vi "Update Position.vi"(8 "error in (no error)":errorcluster, 10 "Diff":cluster{"x":i16, "y":i16}, 11 "Line Border in":refnum<class "Line Border.lvclass">) -> (0 "error out":errorcluster, 1 "EndPoint":cluster{"x":i16, "y":i16}, 2 "StartPoint":cluster{"x":i16, "y":i16}, 3 "Line Border out":refnum<class "Line Border.lvclass">)   [LabVIEW 2015, in "Line Border.lvclass"]
uses:
  Line Border.lvclass
  Scalable Border/Scalable Border.lvclass/Scalable Border.ctl
  Line Border.lvclass/Line Border.ctl
  Scalable Border/Scalable Border.lvclass
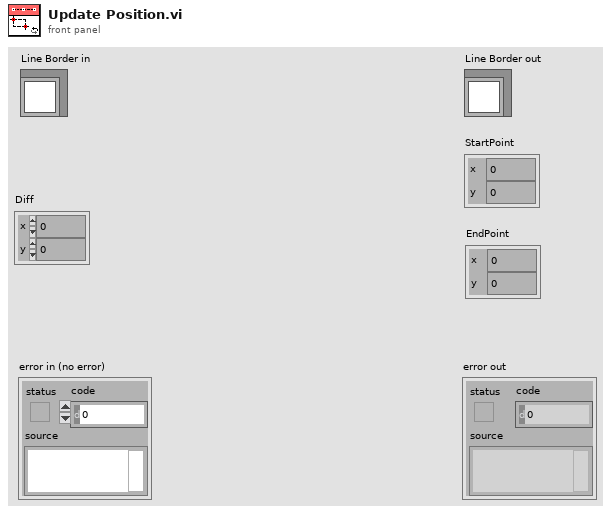
[diagram p1: front panel]
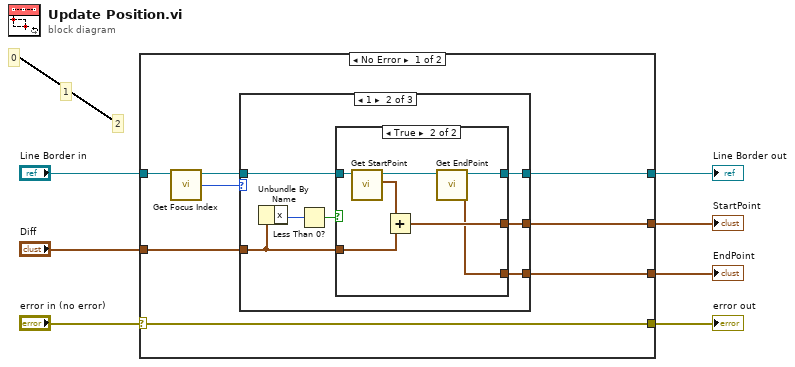
[diagram p0: block diagram]
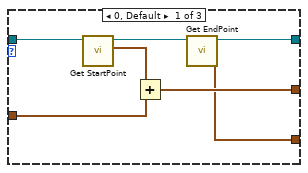
[diagram p2: hidden frame]
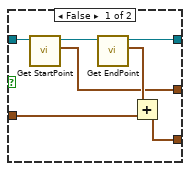
[diagram p3: hidden frame]
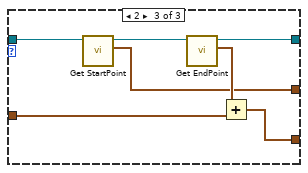
[diagram p4: hidden frame]
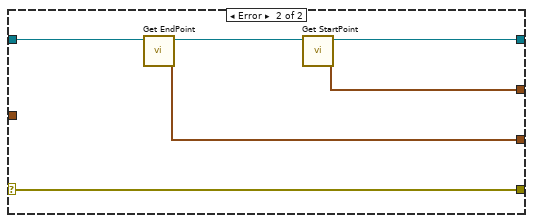
[diagram p5: hidden frame]
diagram:
  # "2"
  # "1"
  # "0"
  n1 = case shown="No Error" "error in (no error)" {
    selector: "error in (no error)" -> [w15 w56]
    tunnel: "Line Border in" -> [w14 w55]
    tunnel: [w11 w54] -> w5
    tunnel: "Diff" -> [w10 _]
    tunnel: [w9 w51] -> w3
    tunnel: [w8 w52] -> w2
    tunnel: [w15 w56] -> w1
    frame No Error {
      n2 = call "Get Focus Index.vi"("Scalable Border in"=w14) -> ("Focus Index"=w13:i8, "Scalable Border out"=w12:refnum<class "Line Border.lvclass">)  [unwired: 8 in, 1 out]
      n3 = case shown="1" w13 {
        tunnel: w12 -> [w22 w29 w50]
        tunnel: [w17 w27 w47] -> w11
        tunnel: w10 -> [w19 w25 w48]
        tunnel: [w18 w28 w44] -> w9
        tunnel: [w16 w26 w45] -> w8
        frame 0, Default {
          n4 = call "Get StartPoint.vi"("Line Border in"=w22) -> ("StartPoint"=w20:cluster{"x":i16, "y":i16}, "Line Border out"=w21:refnum<class "Line Border.lvclass">)  [unwired: 8 in, 1 out]
          n5 = Add(x=w20, y=w19) -> (x+y=w18:cluster{"x":i16, "y":i16})
          n6 = call "Get EndPoint.vi"("Line Border in"=w21) -> ("EndPoint"=w16:cluster{"x":i16, "y":i16}, "Line Border out"=w17:refnum<class "Line Border.lvclass">)  [unwired: 8 in, 1 out]
        }
        frame 1 {
          n7 = Unbundle By Name(w25) -> ("x"=w24:i16)
          n8 = Less Than 0?(x=w24) -> (x < 0?=w23:bool)
          n9 = case shown="True" w23 {
            tunnel: w29 -> [w34 w43]
            tunnel: [w32 w40] -> w28
            tunnel: [w33 w39] -> w27
            tunnel: [w30 w38] -> w26
            tunnel: w25 -> [w31 w37]
            frame False {
              n10 = call "Get StartPoint.vi"("Line Border in"=w34) -> ("StartPoint"=w32:cluster{"x":i16, "y":i16}, "Line Border out"=w36:refnum<class "Line Border.lvclass">)  [unwired: 8 in, 1 out]
              n11 = call "Get EndPoint.vi"("Line Border in"=w36) -> ("EndPoint"=w35:cluster{"x":i16, "y":i16}, "Line Border out"=w33:refnum<class "Line Border.lvclass">)  [unwired: 8 in, 1 out]
              n12 = Add(x=w35, y=w31) -> (x+y=w30:cluster{"x":i16, "y":i16})
            }
            frame True {
              n13 = call "Get StartPoint.vi"("Line Border in"=w43) -> ("StartPoint"=w41:cluster{"x":i16, "y":i16}, "Line Border out"=w42:refnum<class "Line Border.lvclass">)  [unwired: 8 in, 1 out]
              n14 = Add(x=w41, y=w37) -> (x+y=w40:cluster{"x":i16, "y":i16})
              n15 = call "Get EndPoint.vi"("Line Border in"=w42) -> ("EndPoint"=w38:cluster{"x":i16, "y":i16}, "Line Border out"=w39:refnum<class "Line Border.lvclass">)  [unwired: 8 in, 1 out]
            }
          }
        }
        frame 2 {
          n16 = call "Get StartPoint.vi"("Line Border in"=w50) -> ("StartPoint"=w44:cluster{"x":i16, "y":i16}, "Line Border out"=w49:refnum<class "Line Border.lvclass">)  [unwired: 8 in, 1 out]
          n17 = call "Get EndPoint.vi"("Line Border in"=w49) -> ("EndPoint"=w46:cluster{"x":i16, "y":i16}, "Line Border out"=w47:refnum<class "Line Border.lvclass">)  [unwired: 8 in, 1 out]
          n18 = Add(x=w46, y=w48) -> (x+y=w45:cluster{"x":i16, "y":i16})
        }
      }
    }
    frame Error {
      n19 = call "Get EndPoint.vi"("Line Border in"=w55) -> ("EndPoint"=w52:cluster{"x":i16, "y":i16}, "Line Border out"=w53:refnum<class "Line Border.lvclass">)  [unwired: 8 in, 1 out]
      n20 = call "Get StartPoint.vi"("Line Border in"=w53) -> ("StartPoint"=w51:cluster{"x":i16, "y":i16}, "Line Border out"=w54:refnum<class "Line Border.lvclass">)  [unwired: 8 in, 1 out]
    }
  }
  "error out" <- w1
  "Line Border out" <- w5
  "EndPoint" <- w2
  "StartPoint" <- w3
